vi "ImgTriggerRotationAcquire.vi"(0 "Image in":refnum<class "Image.lvclass">, 5 "TabName":string="TabControl", 7 "Page":i32=1, 9 "Control Name":string="Aquire AngleScan", 11 "error in (no error)":errorcluster, 12 "relative vi path":string="RotationProgram\\RotationApplication.vi") -> (4 "Image out":refnum<class "Image.lvclass">, 15 "error out":errorcluster)   [LabVIEW 2012, in "Image.lvclass"]
uses:
  classes/Image.lvclass
  classes/Image.lvclass/Image.ctl
panel:
  out "VI out":refnum<vi>
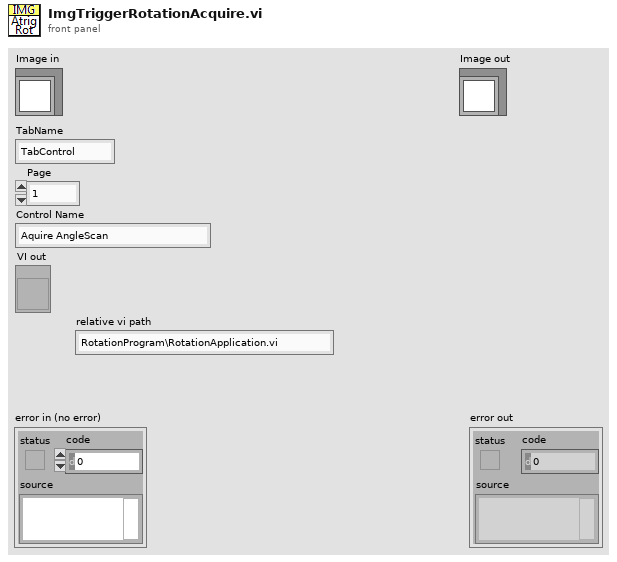
[diagram p1: front panel]
types:
  T1 = typedef "ScanMode.ctl" = enum16{"None", "Continuous", "Point Scan (CH3 cursor)", "Point Scan Move (CH3 cursor)", "Grab", "Grab Move Stage", "Grab Move Z-stage", "Cont. Move Z-stage", "Spec Move Stage", "Spec Move Cont", "Surf Calib"}
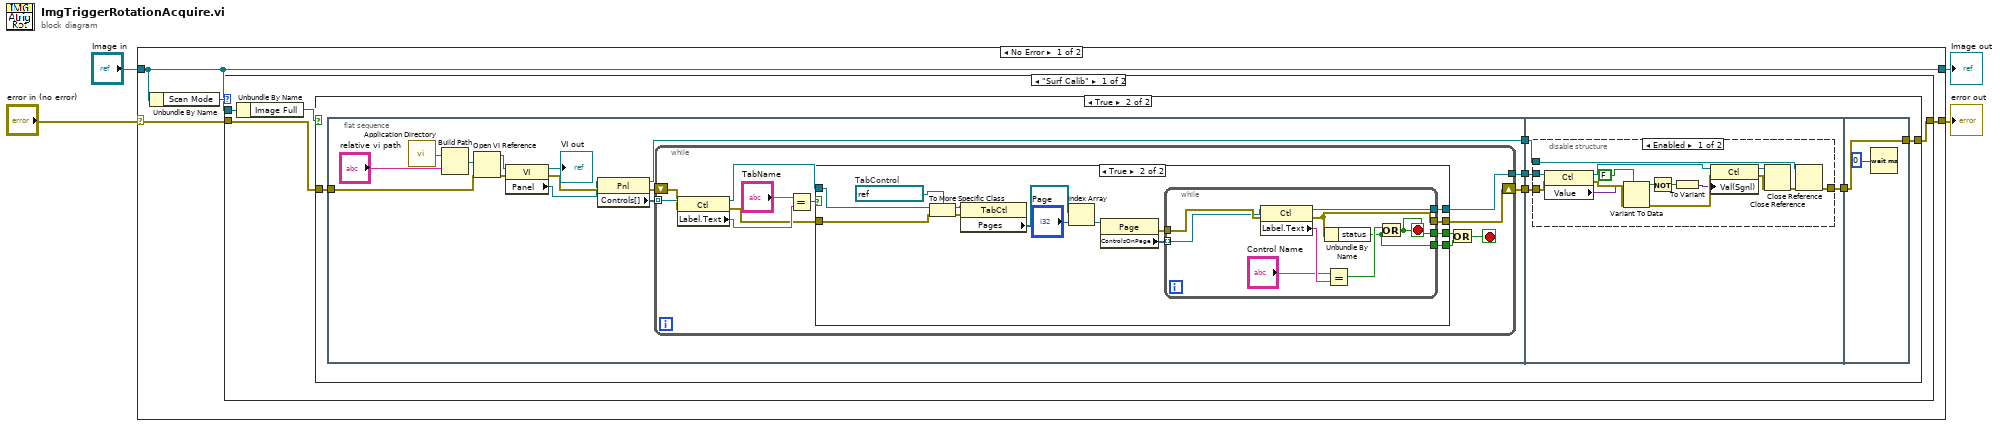
[diagram p0: block diagram]
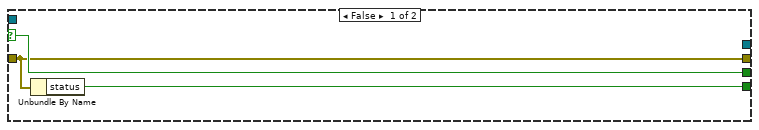
[diagram p3: hidden frame]
diagram:
  n1 = case shown="No Error" "error in (no error)" {
    selector: "error in (no error)" -> [w8 w94]
    tunnel: [w7 w94] -> w3
    tunnel: [w5 w93] -> w1
    tunnel: "Image in" -> [w5 w93]
    frame No Error {
      n2 = Unbundle By Name(w5) -> ("Scan Mode"=w6:T1)
      n3 = case shown="\"Surf Calib\"" w6 {
        tunnel: w8 -> [w12 w92]
        tunnel: [w11 w92] -> w7
        tunnel: w5 -> [w10 _]
        frame "Surf Calib" {
          n4 = Unbundle By Name(w10) -> ("Image Full"=w9:bool)
          n5 = case shown="True" w9 {
            tunnel: w12 -> [_ w18]
            tunnel: [_ w14] -> w11
            frame False {
            }
            frame True {
              n6 = flat-sequence {
                tunnel: w18 -> [w23]
                tunnel: [w21] -> w17
                tunnel: [w20] -> w16
                tunnel: [w19] -> w15
                tunnel: w17 -> [w74]
                tunnel: w16 -> [w73]
                tunnel: w15 -> [w72]
                tunnel: [w71] -> w13
                tunnel: [w90] -> w14
                tunnel: w13 -> [w90]
                frame #0 {
                  n7 = call <vilib>:"Application Directory.vi"() -> ("Application Directory"=w27:path)
                  n8 = Build Path(base path=w27, name or relative path="relative vi path") -> (appended path=w26:path)
                  n9 = Open VI Reference(vi path=w26, error in (no error)=w23) -> (vi reference=w25:refnum<vi>, error out=w24:errorcluster)  [unwired: 4 in]
                  n10 = property class="VI"(reference=w25, error in=w24) -> (reference out=→"VI out":refnum<vi>, error out=w31:errorcluster, "Panel"=w28:refnum<vi>)
                  n11 = property class="Pnl"(reference=w28, error in=w31) -> (reference out=w21:refnum<vi>, error out=w32:errorcluster, "Controls[]"=w29:refnum<vi>[])
                  n12 = while {
                    tunnel: w29 -> [w44] mode=indexing
                    tunnel: [w41] -> w20
                    shift-right: [w38] -> w19
                    shift-left: w32 -> [w42]
                    stop <- w39 stop-if-true
                    n13 = property class="Ctl"(reference=w44, error in=w42) -> (reference out=w35:refnum<vi>, error out=w34:errorcluster, "Label.Text"=w43:string)
                    n14 = Equal?(x="TabName", y=w43) -> (x = y?=w40:bool)
                    n15 = case shown="True" w40 {
                      selector: w40 -> [w47 _]
                      tunnel: [_ w61] -> w41
                      tunnel: [w47 w60] -> w36
                      tunnel: [w46 w59] -> w38
                      tunnel: w35 -> [_ w54]
                      tunnel: w34 -> [w46 w52]
                      tunnel: [w45 w48] -> w33
                      frame False {
                        n16 = Unbundle By Name(w46) -> ("status"=w45:bool)
                      }
                      frame True {
                        w55 = refnum<vi> refnum  # TabControl
                        n17 = To More Specific Class(target class=w55, reference=w54, error in=w52) -> (specific class reference=w50:refnum<vi>, error out=w51:errorcluster)
                        n18 = property class="TabCtl"(reference=w50, error in=w51) -> ("Pages"=w53:refnum<vi>[])  [unwired: 2 out]
                        n19 = Index Array(array=w53, index="Page") -> (element=w49:refnum<vi>)
                        n20 = property class="Page"(reference=w49) -> (error out=w57:errorcluster, "ControlsOnPage"=w58:refnum<vi>[])  [unwired: 1 in, 1 out]
                        n21 = while {
                          tunnel: [w70] -> w61
                          tunnel: [w68] -> w60
                          tunnel: w57 -> [w67]
                          tunnel: [w66] -> w59
                          tunnel: w58 -> [w65] mode=indexing
                          tunnel: [w62] -> w48
                          stop <- w68 stop-if-true
                          n22 = property class="Ctl"(reference=w65, error in=w67) -> (reference out=w70:refnum<vi>, error out=w66:errorcluster, "Label.Text"=w64:string)
                          n23 = Unbundle By Name(w66) -> ("status"=w62:bool)
                          n24 = Equal?(x="Control Name", y=w64) -> (x = y?=w69:bool)
                          n25 = Or(x=w69, y=w62) -> (x .or. y?=w68:bool)
                        }
                      }
                    }
                    n26 = Or(x=w36, y=w33) -> (x .or. y?=w39:bool)
                  }
                }
                frame #1 {
                  n27 = disable-structure shown="Enabled" {
                    disable-tunnel: w74 -> [w89 _]
                    disable-tunnel: w73 -> [w77 _]
                    disable-tunnel: [w76 _] -> w71
                    disable-tunnel: w72 -> [w75 _]
                    frame Enabled {
                      n28 = property class="Ctl"(reference=w77, error in=w75) -> (reference out=w78:refnum<vi>, error out=w84:errorcluster, "Value"=w80:variant)
                      n29 = Variant To Data(error in=w84, type=FALSE ("Push Other VI's Button 2"), Variant=w80) -> (data=w83:bool, error out=w85:errorcluster)
                      n30 = Not(x=w83) -> (.not. x?=w82:bool)
                      n31 = To Variant(anything=w82) -> (Variant=w79:variant)
                      n32 = property class="Ctl"(reference=w78, error in=w85, "Val(Sgnl)"=w79) -> (reference out=w88:refnum<vi>, error out=w87:errorcluster)
                      n33 = Close Reference(reference=w88, error in (no error)=w87) -> (error out=w86:errorcluster)
                      n34 = Close Reference(reference=w89, error in (no error)=w86) -> (error out=w76:errorcluster)
                    }
                    frame Disabled {
                    }
                  }
                }
                frame #2 {
                  n35 = Wait (ms)(milliseconds to wait=u32 0) -> ()  [unwired: 1 out]
                }
              }
            }
          }
        }
        frame "None", Default {
        }
      }
    }
    frame Error {
    }
  }
  "error out" <- w3
  "Image out" <- w1
